vi "PostUUT_Action.vi"(7 "Slot":T3, 8 "error in":errorcluster, 10 "TestResult":bool, 11 "GuiRef":T1={"StringOut"=refnum, "AbortOnFail"=refnum, "SN"=refnum, "SN_Length"=refnum, "TestResult"=refnum, "CycleTime"=refnum, "ErrorCode"=refnum, "UUTStatus"=refnum, "DataBaseEnable?"=refnum, "DUTModel"=refnum, "FixtureID"=refnum, "OperatorID"=refnum, "SNReady"=refnum, "StopSlot"=refnum, "NextStep"=refnum, "PassYeild"=refnum, "Failed"=refnum, "Passed"=refnum, "Tested"=refnum, "TestItemsCtl"={"StepName"="", "TestEnable"=FALSE, "LoopCount"=0, "StopOnFail"=FALSE, "Index"=0, "TestName"="", "通道"="", "参数"="", "TimeStart"=0}, "ProcessBar"=refnum, "Slot"=enum."Slot1", "Row"=3, "States"=refnum, "TestMode"=refnum, "循环次数-DUT"=refnum, "波形图"=refnum, "产品型号"=refnum, "子面板"=refnum, "测试失败项目"=refnum, "测试结果"=refnum, "DUT"=refnum, "Starttime"=refnum, "SlotReady"=refnum, "版本信息"=refnum}) -> (0 "error out":errorcluster)   [LabVIEW 2013]
uses:
  SystemCode/SysControl/Slot.ctl
  Controls/DAQConfig.ctl
  SystemCode/SysControl/Reference.ctl
  SystemCode/SysControl/TestItemsCTL.ctl
panel:
  out "DAQConfig":T4={"DIO"=[["钥匙keyin", "Dev2/port0/line0", "H", "DI"], ["遥控解锁", "Dev2/port0/line1", "H", "DI"], ["后背门", "Dev2/port0/line2", "H", "DI"], ["车门1", "Dev2/port0/line3", "H", "DI"]], "AO"=[["钥匙keyin", "Dev2/port0/line0", "H", "DI"], ["遥控解锁", "Dev2/port0/line1", "H", "DI"], ["后背门", "Dev2/port0/line2", "H", "DI"], ["车门1", "Dev2/port0/line3", "H", "DI"]], "AI"=[["钥匙keyin", "Dev2/port0/line0", "H", "DI"], ["遥控解锁", "Dev2/port0/line1", "H", "DI"], ["后背门", "Dev2/port0/line2", "H", "DI"], ["车门1", "Dev2/port0/line3", "H", "DI"]]}
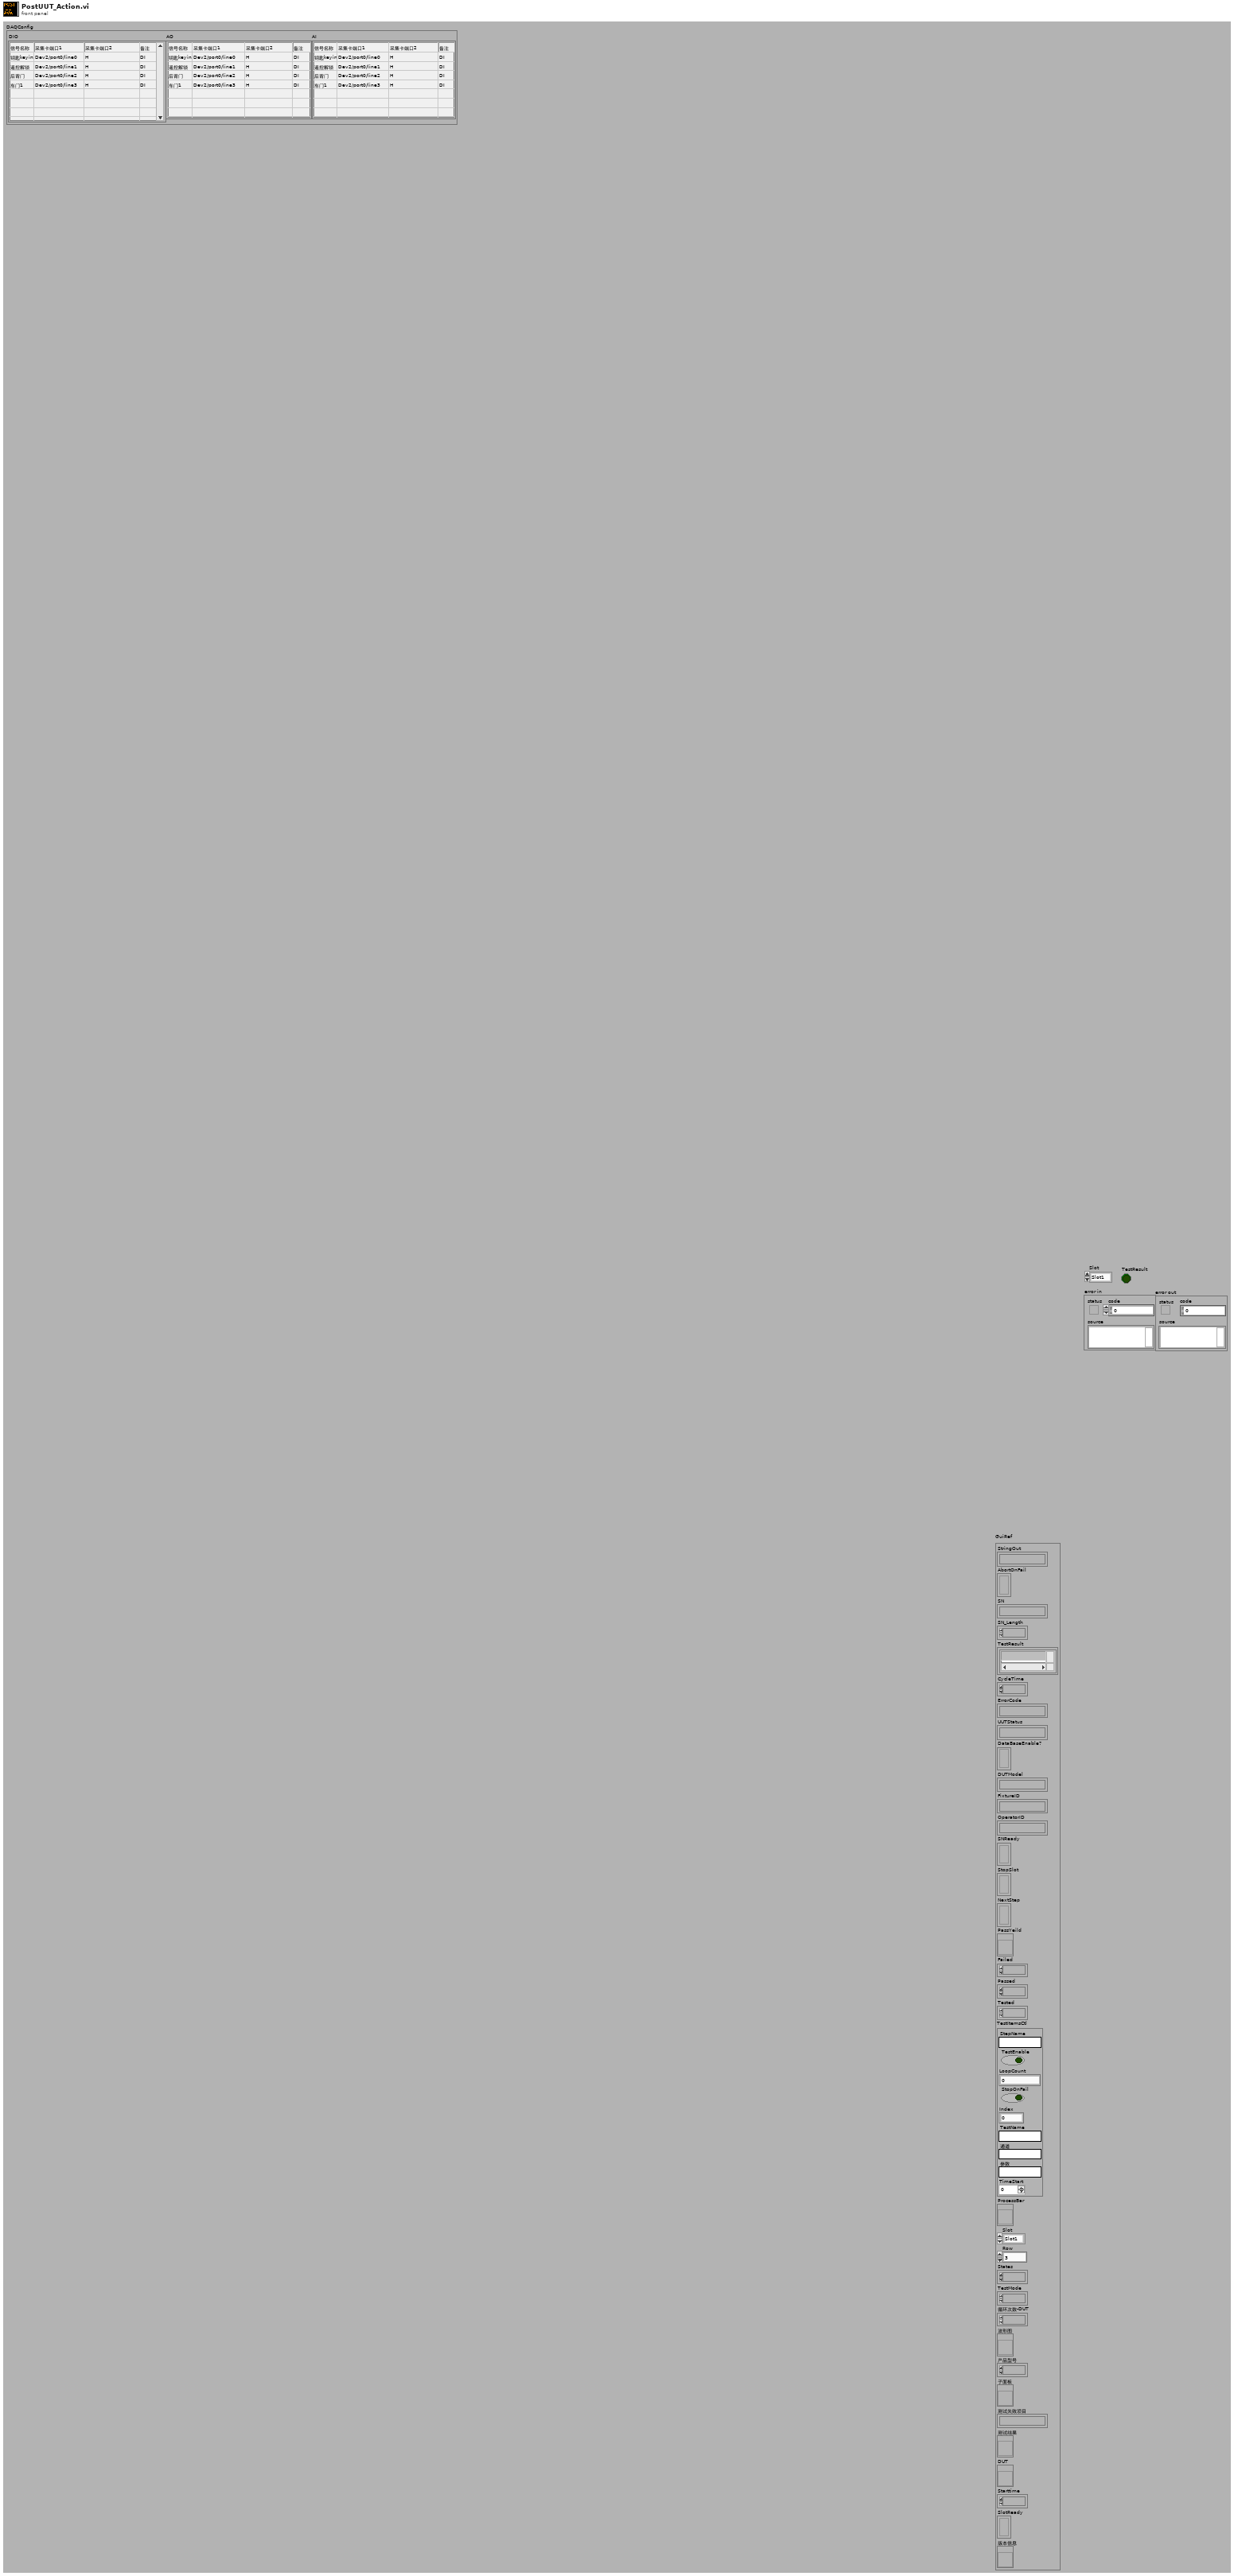
[diagram p1: front panel]
types:
  T1 = typedef "Reference.ctl" = cluster{"StringOut":refnum<vi>, "AbortOnFail":refnum<vi>, "SN":refnum<vi>, "SN_Length":refnum<vi>, "TestResult":refnum<vi>, "CycleTime":refnum<vi>, "ErrorCode":refnum<vi>, "UUTStatus":refnum<vi>, "DataBaseEnable?":refnum<vi>, "DUTModel":refnum<vi>, "FixtureID":refnum<vi>, "OperatorID":refnum<vi>, "SNReady":refnum<vi>, "StopSlot":refnum<vi>, "NextStep":refnum<vi>, "PassYeild":refnum<vi>, "Failed":refnum<vi>, "Passed":refnum<vi>, "Tested":refnum<vi>, "TestItemsCtl":T2, "ProcessBar":refnum<vi>, "Slot":T3, "Row":u32, "States":refnum<vi>, "TestMode":refnum<vi>, "循环次数-DUT":refnum<vi>, "波形图":refnum<vi>, "产品型号":refnum<vi>, "子面板":refnum<vi>, "测试失败项目":refnum<vi>, "测试结果":refnum<vi>, "DUT":refnum<vi>, "Starttime":refnum<vi>, "SlotReady":refnum<vi>, "版本信息":refnum<vi>}
  T2 = typedef "TestItemsCTL.ctl" = cluster{"StepName":string, "TestEnable":bool, "LoopCount":i32, "StopOnFail":bool, "Index":u32, "TestName":string, "通道":string, "参数":string, "TimeStart":u32}
  T3 = typedef "Slot.ctl" = enum16{"Slot1", "Slot2", "Slot3", "Slot4"}
  T4 = typedef "DAQConfig.ctl" = cluster{"DIO":string[][], "AO":string[][], "AI":string[][]}
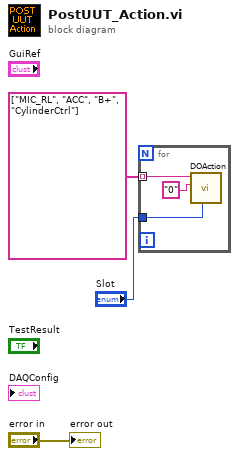
[diagram p0: block diagram]
diagram:
  n1 = for "For循环" {
    tunnel: "Slot" -> [w5]
    tunnel: string[] ["MIC_RL", "ACC", "B+", "CylinderCtrl"] -> [w4] mode=indexing
    n2 = call "DOAction.vi"("Slot"=w5, "State"="0", "CH"=w4) -> ()  [unwired: 8 in, 1 out]
  }
  "error out" <- "error in"
